vi "Globals.vi"() -> ()   [LabVIEW 2017, in "nifxpmath_SinhAndCosh.xnode"]
uses:
  <vilib>/rvi/FXPMathLib/FxpSinhAndCosh/XNode/nifxpmath_SinhAndCosh.xnode
panel:
  out "SmallIcon w/ 4Wire":picture
  in  "Term C Name":string="cosh(x)"
  in  "Term S Name":string="sinh(x)"
  in  "Term Z Name":string="x"
  out "SmallIcon":picture
  out "NormalBanner":picture
  in  "Term C ID":string="TERM_C"
  in  "Term S ID":string="TERM_S"
  in  "Term Z ID":string="TERM_Z"
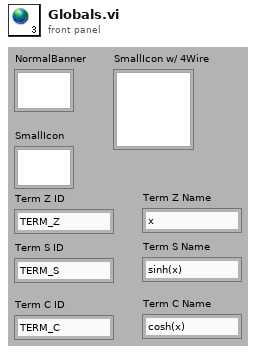
[diagram p1: front panel]
diagram:
